vi "Create User Event.vi"(8 "Error In":errorcluster) -> (0 "Error Out":errorcluster, 3 "User Event Reference":T1)   [LabVIEW 2023, in "QSM - IODocs.lvlib"]
doc: "This VI creates the user event for the Queued Message Handler template."
uses:
  QSM - IODocs.lvlib
  Controls/User Event Reference.ctl
  Controls/User Event Type.ctl
  Controls/Event Handler Message.ctl
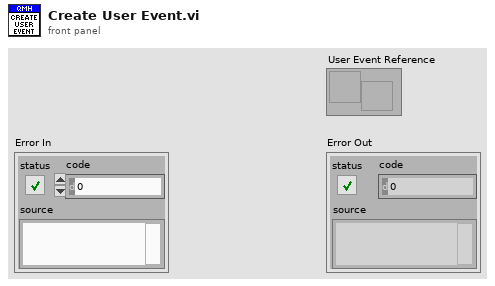
[diagram p1: front panel]
types:
  T1 = typedef "QSM - IODocs.lvlib/User Event Reference.ctl" = refnum<user-event>
  T2 = typedef "QSM - IODocs.lvlib/User Event Type.ctl" = cluster{"Event Handler Message":T3, "Data":variant}
  T3 = typedef "QSM - IODocs.lvlib/Event Handler Message.ctl" = enum16{"Exit"}
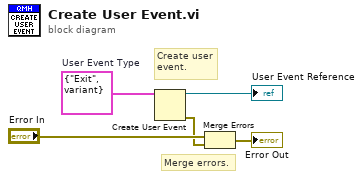
[diagram p0: block diagram]
diagram:
  w5 = T2 {"Event Handler Message"=enum."Exit", "Data"=variant}  # User Event Type
  # "Merge errors."
  # "Create user\nevent."
  n1 = Create User Event(user event datatype=w5) -> (user event=→"User Event Reference":refnum<user-event>, error out=w2:errorcluster)  [unwired: 1 in]
  n2 = Merge Errors("Error In", w2) -> (→"Error Out":errorcluster)
